vi "subtract background.vi"(8 "error in (no error)":errorcluster, 11 "Thorcam in":refnum<class "Thorcam.lvclass">) -> (0 "error out":errorcluster, 3 "Thorcam out":refnum<class "Thorcam.lvclass">)   [LabVIEW 2012, in "Thorcam.lvclass"]
uses:
  Thorcam.lvclass
  Thorcam.lvclass/Thorcam.ctl
  <vilib>/vision/NI_Vision_Development_Module.lvlib
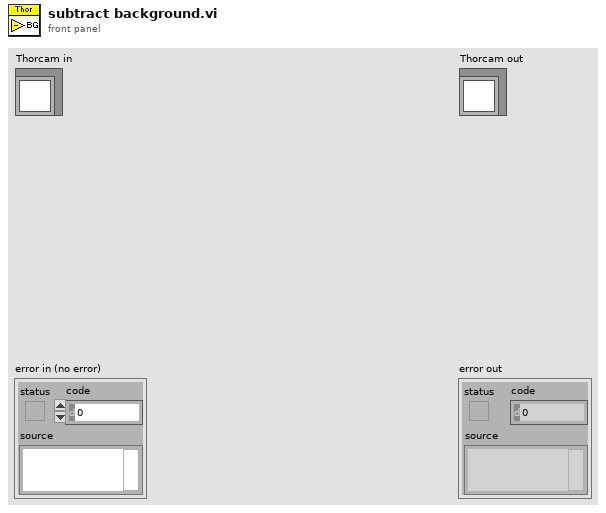
[diagram p1: front panel]
types:
  T1 = typedef "IMAQ Image.ctl" = refnum<image>
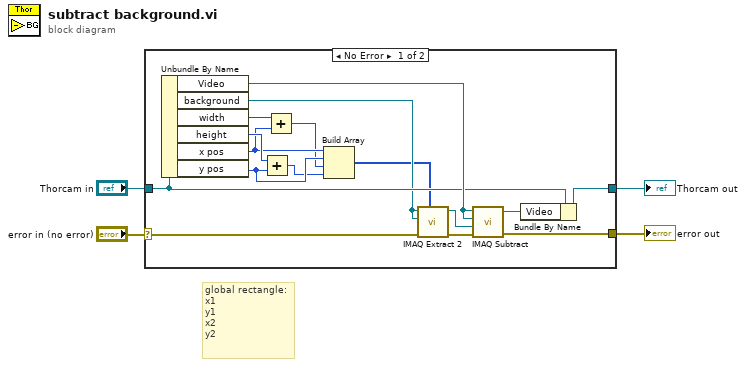
[diagram p0: block diagram]
diagram:
  # "global rectangle:\nx1\ny1\nx2\ny2"
  n1 = case shown="No Error" "error in (no error)" {
    selector: "error in (no error)" -> [w15 w22]
    tunnel: [w16 w22] -> w3
    tunnel: [w18 w21] -> w1
    tunnel: "Thorcam in" -> [w19 w21]
    frame No Error {
      n2 = Unbundle By Name(w19) -> ("Video"=w20:T1, "background"=w7:T1, "width"=w13:i32, "height"=w12:i32, "x pos"=w11:i32, "y pos"=w10:i32)
      n3 = Add(x=w12, y=w10) -> (x+y=w8:i32)
      n4 = Add(x=w13, y=w11) -> (x+y=w9:i32)
      n5 = Build Array(w11, w10, w9, w8) -> (w5:i32[])
      n6 = call "IMAQ Extract 2"("Optional Rectangle"=w5, "error in (no error)"=w15, "Image Dst"=w7, "Image Src"=w7) -> ("error out"=w14:errorcluster, "Image Dst Out"=w6:T1)  [unwired: 6 in]
      n7 = call "IMAQ Subtract"("Image Src A"=w20, "Image Dst"=w20, "Image Src B"=w6, "error in (no error)"=w14) -> ("Image Dst Out"=w17:T1, "error out"=w16:errorcluster)  [unwired: 3 in]
      n8 = Bundle By Name(cluster=w19, "Video"=w17) -> (w18:refnum<class "Thorcam.lvclass">)
    }
    frame Error {
    }
  }
  "error out" <- w3
  "Thorcam out" <- w1
